vi "Main Host Comms Commands.vi"(8 "error in":errorcluster, 10 "main queue":refnum<queue>, 11 "tcp in":refnum<k5>) -> (0 "error out":errorcluster, 2 "processed?":bool, 3 "tcp out":refnum<k5>)   [LabVIEW 2019]
uses:
  RT Controls/Main Process Commands.ctl
  RT Controls/Main Command Events.ctl
panel:
  out "error msg":string
  out "cmd":string
  out "subcmd":string
  out "full cmd":string
  out "single cmd?":bool
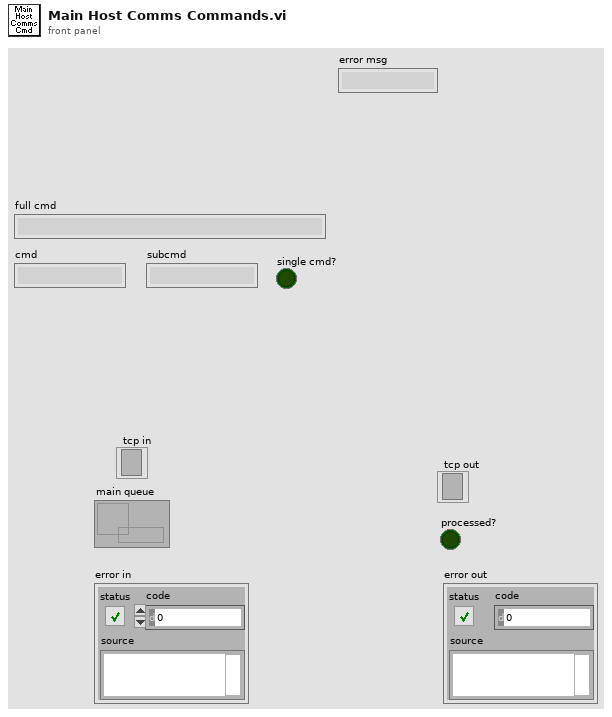
[diagram p1: front panel]
types:
  T1 = enum16{"Standard", "Buffered", "CRLF", "Immediate"}
  T2 = typedef "Main Process Commands.ctl" = cluster{"Commands":T3, "Value":variant}
  T3 = typedef "Main Command Events.ctl" = enum16{"Idle", "FullStop", "MainReadConfig", "MainWriteConfig", "OpenUpper", "CloseUpper", "OpenLower", "CloseLower", "SetWatchdogInt", "EnCloudShutDn", "DisCloudShutDn", "SetRainDelay", "EnAutoShutDn", "DisAutoShutDn", "SetRevDelay", "RotToAz", "RotLeft", "RotRight", "RotToHome", "DefineHomePos", "SetHSThres", "SetEncCounts", "SyncClose", "SyncOpen", "SetAZTimLim", "SetAZTol", "AZEncPositive", "AZEncNegative", "RotToCenter"}
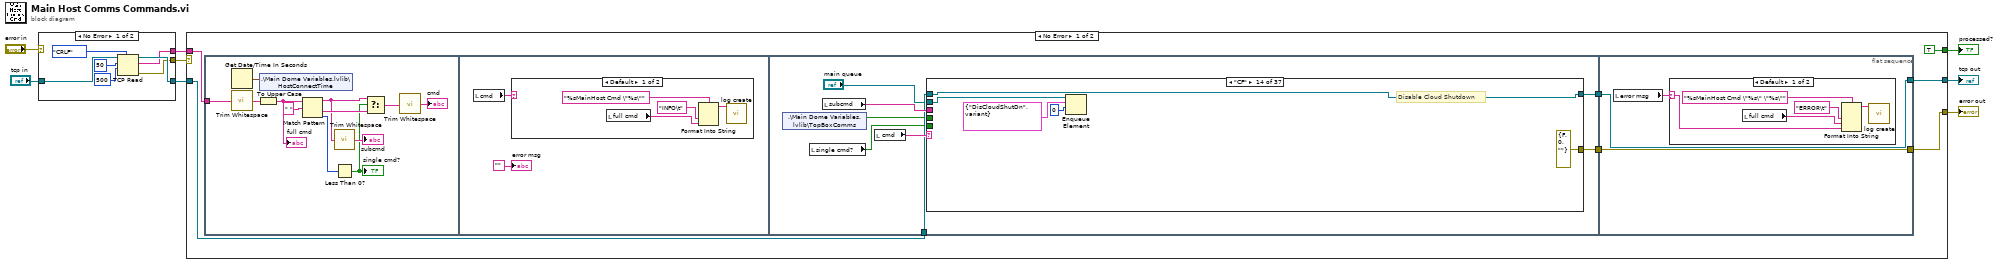
[diagram p0: block diagram]
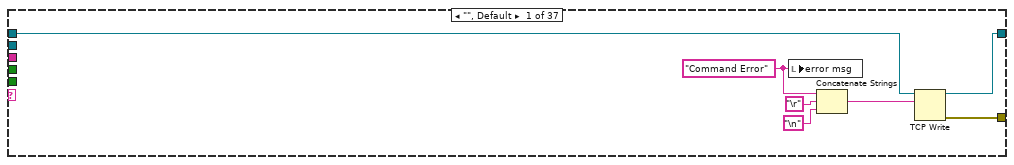
[diagram p3: hidden frame]
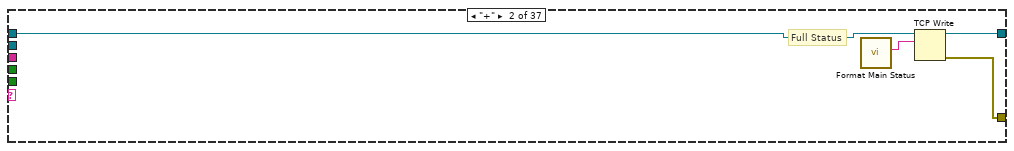
[diagram p4: hidden frame]
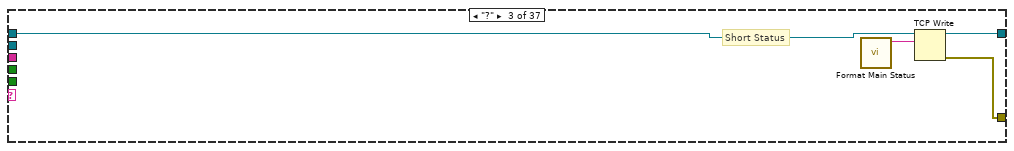
[diagram p5: hidden frame]
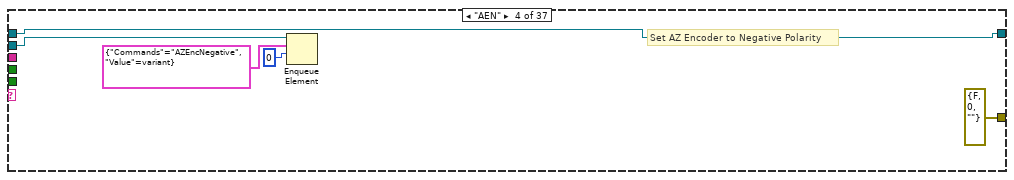
[diagram p6: hidden frame]
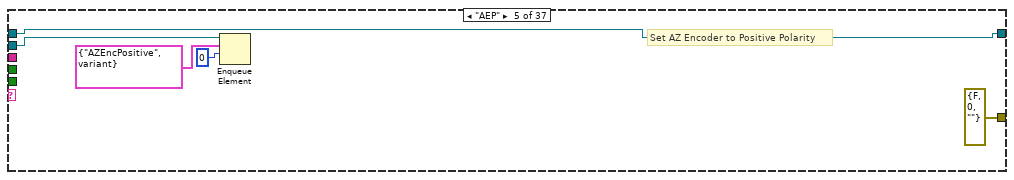
[diagram p7: hidden frame]
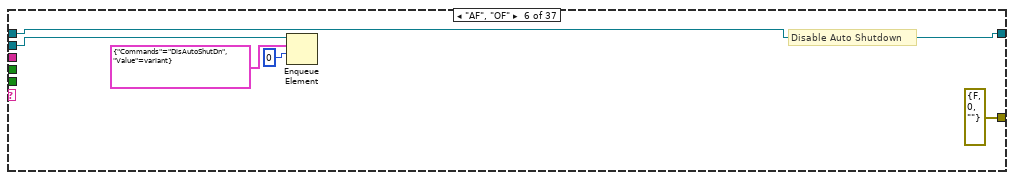
[diagram p8: hidden frame]
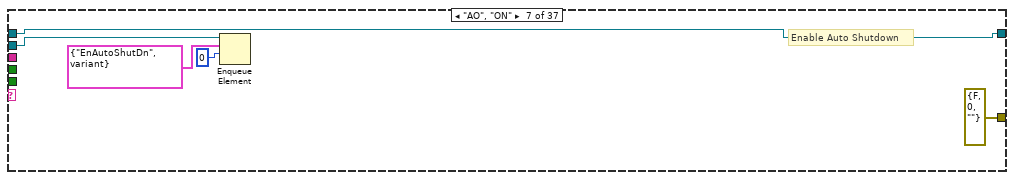
[diagram p9: hidden frame]
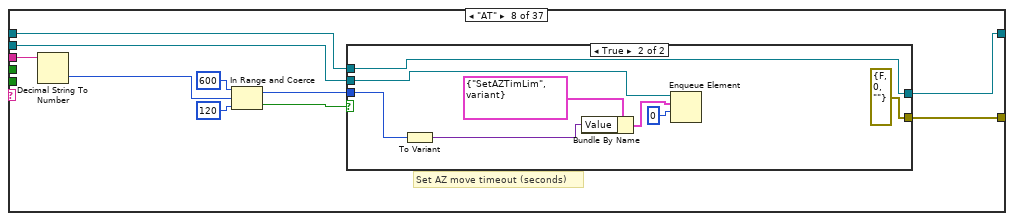
[diagram p10: hidden frame]
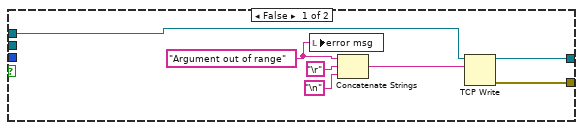
[diagram p11: hidden frame]
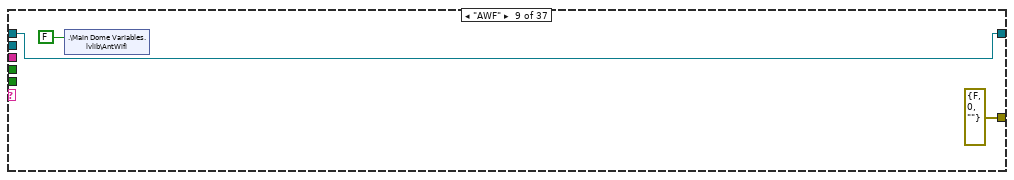
[diagram p12: hidden frame]
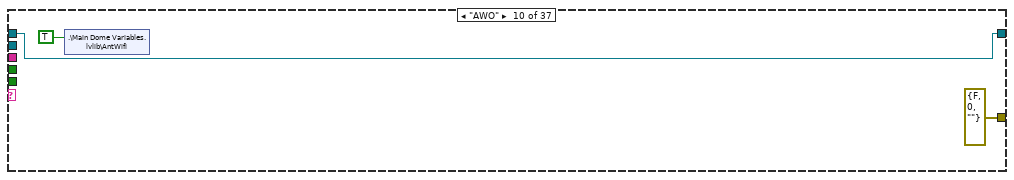
[diagram p13: hidden frame]
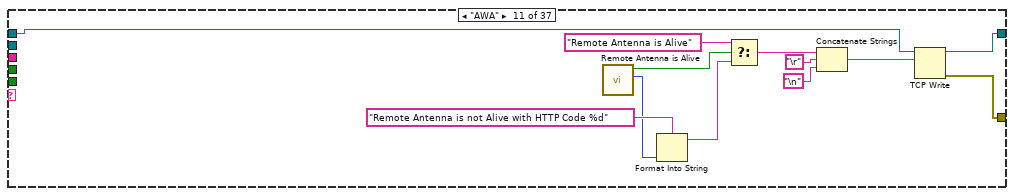
[diagram p14: hidden frame]
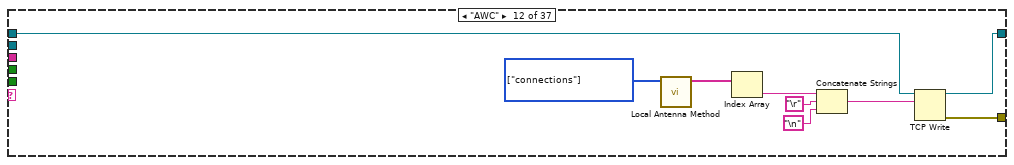
[diagram p15: hidden frame]
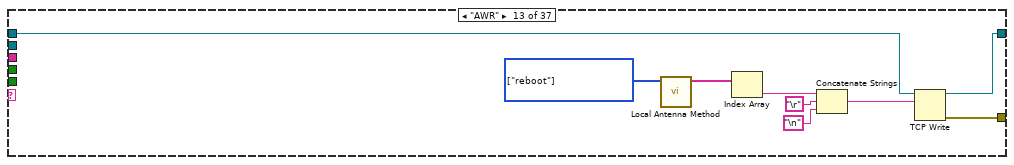
[diagram p16: hidden frame]
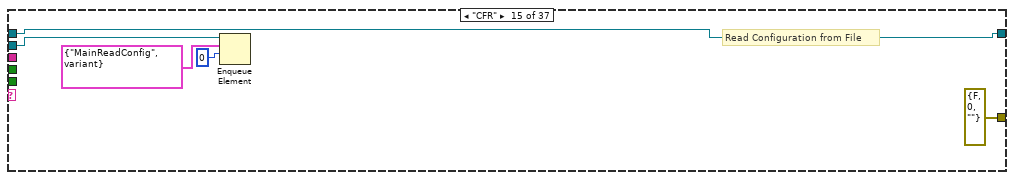
[diagram p17: hidden frame]
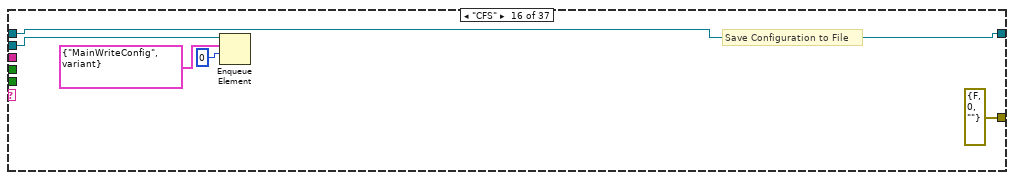
[diagram p18: hidden frame]
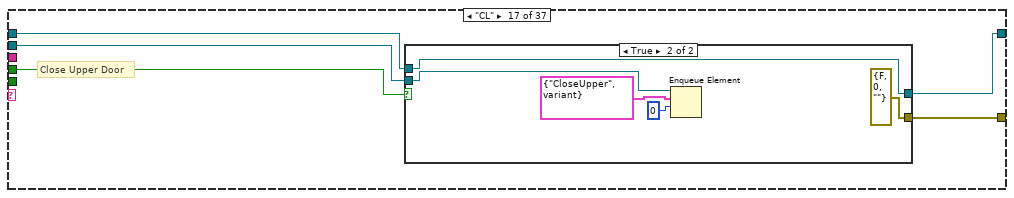
[diagram p19: hidden frame]
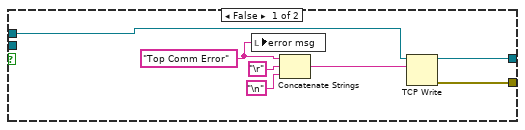
[diagram p20: hidden frame]
diagram:
  n1 = case shown="No Error" "error in" {
    selector: "error in" -> [_ w16]
    tunnel: "tcp in" -> [w15 w18]
    tunnel: [w11 w18] -> w6
    tunnel: [w10 "" ("data out")] -> w7
    tunnel: [w9 w16] -> w8
    frame No Error {
      n2 = TCP Read(connection ID=w15, bytes to read=50, 7:T1."CRLF" ("mode (standard)"), 9:500 ("timeout ms (25000)")) -> (connection ID out=w11:refnum<k5>, data out=w10:string, error out=w9:errorcluster)  [unwired: 1 in]
    }
    frame Error {
    }
  }
  n3 = case shown="No Error" w8 {
    selector: w8 -> [_ w570]
    tunnel: w7 -> [w24 _]
    tunnel: w6 -> [w23 w567]
    tunnel: [w21 w567] -> w2
    tunnel: [w22 w569] -> w3
    tunnel: [TRUE FALSE] -> w1
    frame No Error {
      n4 = flat-sequence {
        tunnel: w24 -> [w28]
        tunnel: w23 -> [w49]
        tunnel: [w48] -> w20
        tunnel: [w47] -> w19
        tunnel: [w560] -> w21
        tunnel: [w561] -> w22
        tunnel: w20 -> [w561]
        tunnel: w19 -> [w560]
        frame #0 {
          n5 = Get Date/Time In Seconds() -> (seconds since 1Jan1904=w26:timestamp)
          n6 = call <vilib>:"Trim Whitespace.vi"("string"=w28) -> ("trimmed string"=w37:string)  [unwired: 1 in]
          n7 = To Upper Case(1:w37) -> (0:w27:string)
          "full cmd" <- w27
          n8 = shared-variable ".\\Main Dome Variables.lvlib\\HostConnectTime"(w26) -> ()  [unwired: 1 in, 1 out]
          n9 = Match Pattern(string=w27, regular expression=" ") -> (before substring=w31:string, after substring=w34:string, offset past match=w35:i32)  [unwired: 1 in, 1 out]
          n10 = call <vilib>:"Trim Whitespace.vi"("string"=w31) -> ("trimmed string"=→"subcmd":string)  [unwired: 1 in]
          n11 = Less Than 0?(x=w35) -> (x < 0?=w29:bool)
          "single cmd?" <- w29
          n12 = Select(t=w31, s=w29, f=w34) -> (s? t:f=w32:string)
          n13 = call <vilib>:"Trim Whitespace.vi"("string"=w32) -> ("trimmed string"=→"cmd":string)  [unwired: 1 in]
        }
        frame #1 {
          n14 = local read "cmd"() -> (w39:string)
          n15 = case shown="Default" w39 {
            frame Default {
              n16 = local read "full cmd"() -> (w40:string)
              n17 = Format Into String(format string="%sMainHost Cmd \"%s\"", "INFO\t" ("input 1"), w40) -> (resulting string=w41:string)  [unwired: 2 in, 1 out]
              n18 = call "log create.vi"("message"=w41) -> ()  [unwired: 11 in]
            }
            frame "+", "?", "HELP" {
            }
          }
          "error msg" <- ""
        }
        frame #2 {
          n19 = shared-variable ".\\Main Dome Variables.lvlib\\TopBoxComms"() -> (w46:bool)  [unwired: 1 in, 1 out]
          n20 = local read "single cmd?"() -> (w45:bool)
          n21 = local read "subcmd"() -> (w51:string)
          n22 = local read "cmd"() -> (w50:string)
          n23 = case shown="\"CF\"" w50 {
            tunnel: w49 -> [w56 w60 w65 w71 w76 w81 w86 w93 w112 w115 w126 w132 w141 w152 w157 w162 w167 w184 w189 w193 w210 w215 w225 w253 w281 w311 w337 w359 w383 w405 w435 w457 w475 w491 w504 w524 w541]
            tunnel: [w58 w62 w66 errorcluster {"status"=FALSE, "code"=0, "source"=""} ("error out") errorcluster {"status"=FALSE, "code"=0, "source"=""} ("error out") errorcluster {"status"=FALSE, "code"=0, "source"=""} ("error out") errorcluster {"status"=FALSE, "code"=0, "source"=""} ("error out") w89 errorcluster {"status"=FALSE, "code"=0, "source"=""} ("error out") errorcluster {"status"=FALSE, "code"=0, "source"=""} ("error out") w118 w130 w139 errorcluster {"status"=FALSE, "code"=0, "source"=""} ("error out") errorcluster {"status"=FALSE, "code"=0, "source"=""} ("error out") errorcluster {"status"=FALSE, "code"=0, "source"=""} ("error out") w164 errorcluster {"status"=FALSE, "code"=0, "source"=""} ("error out") errorcluster {"status"=FALSE, "code"=0, "source"=""} ("error out") w192 w208 errorcluster {"status"=FALSE, "code"=0, "source"=""} ("error out") w222 w250 w279 w309 w334 w358 w380 w404 w432 w455 w472 errorcluster {"status"=FALSE, "code"=0, "source"=""} ("error out") w502 w522 w540] -> w48
            tunnel: [w57 w61 w64 w71 w76 w81 w86 w90 w112 w115 w125 w131 w140 w152 w157 w162 w165 w184 w189 w191 w209 w215 w223 w251 w280 w310 w335 w357 w381 w403 w433 w456 w473 w491 w503 w521 w539] -> w47
            tunnel: w51 -> [_ _ _ _ _ _ _ w92 _ _ _ _ _ _ _ _ _ _ _ _ _ _ w221 w249 w278 w304 w333 _ w379 w410 w431 _ _ _ w497 _ w543]
            tunnel: w45 -> [_ _ _ _ _ _ _ _ _ _ _ _ _ _ _ _ _ _ _ _ _ _ w218 w246 w274 w301 w330 _ w376 _ w428 _ _ _ w494 _ _]
            tunnel: w46 -> [_ _ _ _ _ _ _ _ _ _ _ _ _ _ _ _ w166 _ _ w194 _ _ _ _ _ _ _ w360 _ _ _ w458 w474 _ _ w523 _]
            tunnel: "main queue" -> [_ _ _ w68 w73 w78 w83 w87 _ _ _ _ _ w148 w154 w159 w163 w181 w186 w190 _ w212 w217 w245 w273 w300 w329 w356 w375 w401 w427 w454 w471 w490 w493 w520 w537]
            frame "", Default {
              w52 = "Command Error" ("data in")
              n24 = local write "error msg"(w52) -> ()
              n25 = Concatenate Strings(w52, "\r", "\n") -> (w53:string)
              n26 = TCP Write(connection ID=w56, data in=w53) -> (connection ID out=w57:refnum<k5>, error out=w58:errorcluster)  [unwired: 2 in, 1 out]
            }
            frame "+" {
              # "Full Status"
              n27 = call "Format Main Status.vi"() -> ("FullStat"=w59:string)  [unwired: 10 in, 1 out]
              n28 = TCP Write(connection ID=w60, data in=w59) -> (connection ID out=w61:refnum<k5>, error out=w62:errorcluster)  [unwired: 2 in, 1 out]
            }
            frame "?" {
              # "Short Status"
              n29 = call "Format Main Status.vi"() -> ("ShortStat"=w63:string)  [unwired: 10 in, 1 out]
              n30 = TCP Write(connection ID=w65, data in=w63) -> (connection ID out=w64:refnum<k5>, error out=w66:errorcluster)  [unwired: 2 in, 1 out]
            }
            frame "AEN" {
              # "Set AZ Encoder to Negative Polarity"
              n31 = Enqueue Element(queue=w68, element=T2 {"Commands"=enum."AZEncNegative", "Value"=variant} ("event data"), timeout in ms (-1)=0) -> ()  [unwired: 1 in, 3 out]
            }
            frame "AEP" {
              # "Set AZ Encoder to Positive Polarity"
              n32 = Enqueue Element(queue=w73, element=T2 {"Commands"=enum."AZEncPositive", "Value"=variant} ("event data"), timeout in ms (-1)=0) -> ()  [unwired: 1 in, 3 out]
            }
            frame "AF", "OF" {
              # "Disable Auto Shutdown"
              n33 = Enqueue Element(queue=w78, element=T2 {"Commands"=enum."DisAutoShutDn", "Value"=variant} ("event data"), timeout in ms (-1)=0) -> ()  [unwired: 1 in, 3 out]
            }
            frame "AO", "ON" {
              # "Enable Auto Shutdown"
              n34 = Enqueue Element(queue=w83, element=T2 {"Commands"=enum."EnAutoShutDn", "Value"=variant} ("event data"), timeout in ms (-1)=0) -> ()  [unwired: 1 in, 3 out]
            }
            frame "AT" {
              # "Set AZ move timeout (seconds)"
              n35 = Decimal String To Number(string=w92) -> (number=w96:i32)  [unwired: 2 in, 1 out]
              n36 = In Range and Coerce(upper limit=600, x=w96, lower limit=120) -> (coerced(x)=w91:i32, In Range?=w94:bool)
              n37 = case shown="True" w94 {
                tunnel: w93 -> [w102 w111]
                tunnel: [w103 errorcluster {"status"=FALSE, "code"=0, "source"=""} ("error out")] -> w89
                tunnel: [w101 w111] -> w90
                tunnel: w91 -> [_ w110]
                tunnel: w87 -> [_ w105]
                frame False {
                  w97 = "Argument out of range" ("data in")
                  n38 = local write "error msg"(w97) -> ()
                  n39 = Concatenate Strings(w97, "\r", "\n") -> (w98:string)
                  n40 = TCP Write(connection ID=w102, data in=w98) -> (connection ID out=w101:refnum<k5>, error out=w103:errorcluster)  [unwired: 2 in, 1 out]
                }
                frame True {
                  n41 = To Variant(anything=w110) -> (Variant=w109:variant)
                  n42 = Bundle By Name(cluster=T2 {"Commands"=enum."SetAZTimLim", "Value"=variant} ("event data"), "Value"=w109) -> (w106:T2)
                  n43 = Enqueue Element(queue=w105, element=w106, timeout in ms (-1)=0) -> ()  [unwired: 1 in, 3 out]
                }
              }
            }
            frame "AWF" {
              n44 = shared-variable ".\\Main Dome Variables.lvlib\\AntWifi"(FALSE ("AntWifi")) -> ()  [unwired: 1 in, 1 out]
            }
            frame "AWO" {
              n45 = shared-variable ".\\Main Dome Variables.lvlib\\AntWifi"(TRUE ("AntWifi")) -> ()  [unwired: 1 in, 1 out]
            }
            frame "AWA" {
              n46 = call "Remote Antenna is Alive.vi"() -> ("http code"=w120:i32, "alive?"=w124:bool)  [unwired: 10 in]
              n47 = Format Into String(format string="Remote Antenna is not Alive with HTTP Code %d", w120) -> (resulting string=w119:string)  [unwired: 2 in, 1 out]
              n48 = Select(t="Remote Antenna is Alive" ("data in"), s=w124, f=w119) -> (s? t:f=w122:string)
              n49 = Concatenate Strings(w122, "\r", "\n") -> (w129:string)
              n50 = TCP Write(connection ID=w126, data in=w129) -> (connection ID out=w125:refnum<k5>, error out=w118:errorcluster)  [unwired: 2 in, 1 out]
            }
            frame "AWC" {
              w138 = enum16{"connections", "reboot"}[] [enum."connections"] items=["connections", "reboot"] ("command (connections)")
              n51 = call "Local Antenna Method.vi"("command"=w138) -> ("out"=w137:string[])  [unwired: 10 in]
              n52 = Index Array(array=w137) -> (element=w133:string)  [unwired: 1 in]
              n53 = Concatenate Strings(w133, "\r", "\n") -> (w136:string)
              n54 = TCP Write(connection ID=w132, data in=w136) -> (connection ID out=w131:refnum<k5>, error out=w130:errorcluster)  [unwired: 2 in, 1 out]
            }
            frame "AWR" {
              w142 = enum16{"connections", "reboot"}[] [enum."reboot"] items=["connections", "reboot"] ("command (connections)")
              n55 = call "Local Antenna Method.vi"("command"=w142) -> ("out"=w147:string[])  [unwired: 10 in]
              n56 = Index Array(array=w147) -> (element=w145:string)  [unwired: 1 in]
              n57 = Concatenate Strings(w145, "\r", "\n") -> (w146:string)
              n58 = TCP Write(connection ID=w141, data in=w146) -> (connection ID out=w140:refnum<k5>, error out=w139:errorcluster)  [unwired: 2 in, 1 out]
            }
            frame "CF" {
              # "Disable Cloud Shutdown"
              n59 = Enqueue Element(queue=w148, element=T2 {"Commands"=enum."DisCloudShutDn", "Value"=variant} ("event data"), timeout in ms (-1)=0) -> ()  [unwired: 1 in, 3 out]
            }
            frame "CFR" {
              # "Read Configuration from File"
              n60 = Enqueue Element(queue=w154, element=T2 {"Commands"=enum."MainReadConfig", "Value"=variant} ("event data"), timeout in ms (-1)=0) -> ()  [unwired: 1 in, 3 out]
            }
            frame "CFS" {
              # "Save Configuration to File"
              n61 = Enqueue Element(queue=w159, element=T2 {"Commands"=enum."MainWriteConfig", "Value"=variant} ("event data"), timeout in ms (-1)=0) -> ()  [unwired: 1 in, 3 out]
            }
            frame "CL" {
              # "Close Upper Door"
              n62 = case shown="True" w166 {
                tunnel: w167 -> [w170 w179]
                tunnel: [w169 w179] -> w165
                tunnel: [w171 errorcluster {"status"=FALSE, "code"=0, "source"=""} ("error out")] -> w164
                tunnel: w163 -> [_ w176]
                frame False {
                  w168 = "Top Comm Error" ("data in")
                  n63 = local write "error msg"(w168) -> ()
                  n64 = Concatenate Strings(w168, "\r", "\n") -> (w172:string)
                  n65 = TCP Write(connection ID=w170, data in=w172) -> (connection ID out=w169:refnum<k5>, error out=w171:errorcluster)  [unwired: 2 in, 1 out]
                }
                frame True {
                  n66 = Enqueue Element(queue=w176, element=T2 {"Commands"=enum."CloseUpper", "Value"=variant} ("event data"), timeout in ms (-1)=0) -> ()  [unwired: 1 in, 3 out]
                }
              }
            }
            frame "CN" {
              # "Send Dome to Encoder Center"
              n67 = Enqueue Element(queue=w181, element=T2 {"Commands"=enum."RotToCenter", "Value"=variant} ("event data"), timeout in ms (-1)=0) -> ()  [unwired: 1 in, 3 out]
            }
            frame "CO" {
              # "Enable Cloud Shutdown"
              n68 = Enqueue Element(queue=w186, element=T2 {"Commands"=enum."EnCloudShutDn", "Value"=variant} ("event data"), timeout in ms (-1)=0) -> ()  [unwired: 1 in, 3 out]
            }
            frame "DN" {
              # "Open Lower Door"
              n69 = case shown="False" w194 {
                tunnel: w193 -> [w196 w206]
                tunnel: [w198 errorcluster {"status"=FALSE, "code"=0, "source"=""} ("error out")] -> w192
                tunnel: [w197 w206] -> w191
                tunnel: w190 -> [_ w202]
                frame False {
                  w195 = "Top Comm Error" ("data in")
                  n70 = local write "error msg"(w195) -> ()
                  n71 = Concatenate Strings(w195, "\r", "\n") -> (w199:string)
                  n72 = TCP Write(connection ID=w196, data in=w199) -> (connection ID out=w197:refnum<k5>, error out=w198:errorcluster)  [unwired: 2 in, 1 out]
                }
                frame True {
                  n73 = Enqueue Element(queue=w202, element=T2 {"Commands"=enum."OpenLower", "Value"=variant} ("event data"), timeout in ms (-1)=0) -> ()  [unwired: 1 in, 3 out]
                }
              }
            }
            frame "HELP" {
              n74 = call "Host Help Text.vi"() -> ("Help Text"=w207:string)  [unwired: 11 in]
              n75 = TCP Write(connection ID=w210, data in=w207) -> (connection ID out=w209:refnum<k5>, error out=w208:errorcluster)  [unwired: 2 in, 1 out]
            }
            frame "HM" {
              # "Send Dome to Home"
              n76 = Enqueue Element(queue=w212, element=T2 {"Commands"=enum."RotToHome", "Value"=variant} ("event data"), timeout in ms (-1)=0) -> ()  [unwired: 1 in, 3 out]
            }
            frame "HS" {
              # "Set High Speed Threshold (deg)"
              n77 = Fract/Exp String To Number(string=w221, default (0 dbl)=-10.0 ("default (0 DBL)")) -> (number=w228:dbl)  [unwired: 2 in, 1 out]
              n78 = In Range and Coerce(upper limit=10.0, x=w228, lower limit=0.0) -> (coerced(x)=w224:dbl, In Range?=w220:bool)
              n79 = Compound Arithmetic op=AND(invert w218, w220) -> (w219:bool)
              n80 = case shown="True" w219 {
                tunnel: w225 -> [w234 w243]
                tunnel: [w235 errorcluster {"status"=FALSE, "code"=0, "source"=""} ("error out")] -> w222
                tunnel: [w233 w243] -> w223
                tunnel: w224 -> [_ w242]
                tunnel: w217 -> [_ w237]
                frame False {
                  w229 = "Argument out of range" ("data in")
                  n81 = local write "error msg"(w229) -> ()
                  n82 = Concatenate Strings(w229, "\r", "\n") -> (w230:string)
                  n83 = TCP Write(connection ID=w234, data in=w230) -> (connection ID out=w233:refnum<k5>, error out=w235:errorcluster)  [unwired: 2 in, 1 out]
                }
                frame True {
                  n84 = To Variant(anything=w242) -> (Variant=w241:variant)
                  n85 = Bundle By Name(cluster=T2 {"Commands"=enum."SetHSThres", "Value"=variant} ("event data"), "Value"=w241) -> (w238:T2)
                  n86 = Enqueue Element(queue=w237, element=w238, timeout in ms (-1)=0) -> ()  [unwired: 1 in, 3 out]
                }
              }
            }
            frame "HZ" {
              # "Define Dome Home Position (degs)"
              n87 = Fract/Exp String To Number(string=w249, default (0 dbl)=-10.0 ("lower limit")) -> (number=w256:dbl)  [unwired: 2 in, 1 out]
              n88 = In Range and Coerce(upper limit=360.0, x=w256, lower limit=0.0) -> (coerced(x)=w252:dbl, In Range?=w247:bool)
              n89 = Compound Arithmetic op=AND(invert w246, w247) -> (w248:bool)
              n90 = case shown="True" w248 {
                tunnel: w253 -> [w262 w271]
                tunnel: [w263 errorcluster {"status"=FALSE, "code"=0, "source"=""} ("error out")] -> w250
                tunnel: [w261 w271] -> w251
                tunnel: w252 -> [_ w270]
                tunnel: w245 -> [_ w265]
                frame False {
                  w257 = "Argument out of range" ("data in")
                  n91 = local write "error msg"(w257) -> ()
                  n92 = Concatenate Strings(w257, "\r", "\n") -> (w258:string)
                  n93 = TCP Write(connection ID=w262, data in=w258) -> (connection ID out=w261:refnum<k5>, error out=w263:errorcluster)  [unwired: 2 in, 1 out]
                }
                frame True {
                  n94 = To Variant(anything=w270) -> (Variant=w269:variant)
                  n95 = Bundle By Name(cluster=T2 {"Commands"=enum."DefineHomePos", "Value"=variant} ("event data"), "Value"=w269) -> (w266:T2)
                  n96 = Enqueue Element(queue=w265, element=w266, timeout in ms (-1)=0) -> ()  [unwired: 1 in, 3 out]
                }
              }
            }
            frame "LF" {
              # "Rotate Dome Left by Degrees"
              n97 = Fract/Exp String To Number(string=w278, default (0 dbl)=-10.0 ("default (0 DBL)")) -> (number=w284:dbl)  [unwired: 2 in, 1 out]
              n98 = In Range and Coerce(upper limit=360.0, x=w284, lower limit=0.0) -> (coerced(x)=w277:dbl, In Range?=w276:bool)
              n99 = Compound Arithmetic op=AND(invert w274, w276) -> (w275:bool)
              n100 = case shown="True" w275 {
                tunnel: w281 -> [w290 w299]
                tunnel: [w291 errorcluster {"status"=FALSE, "code"=0, "source"=""} ("error out")] -> w279
                tunnel: [w289 w299] -> w280
                tunnel: w277 -> [_ w298]
                tunnel: w273 -> [_ w292]
                frame False {
                  w285 = "Argument out of range" ("data in")
                  n101 = local write "error msg"(w285) -> ()
                  n102 = Concatenate Strings(w285, "\r", "\n") -> (w286:string)
                  n103 = TCP Write(connection ID=w290, data in=w286) -> (connection ID out=w289:refnum<k5>, error out=w291:errorcluster)  [unwired: 2 in, 1 out]
                }
                frame True {
                  n104 = To Variant(anything=w298) -> (Variant=w297:variant)
                  n105 = Bundle By Name(cluster=T2 {"Commands"=enum."RotLeft", "Value"=variant} ("event data"), "Value"=w297) -> (w293:T2)
                  n106 = Enqueue Element(queue=w292, element=w293, timeout in ms (-1)=0) -> ()  [unwired: 1 in, 3 out]
                }
              }
            }
            frame "LM" {
              # "Set Encoder Counts in 360 deg"
              n107 = Fract/Exp String To Number(string=w304) -> (number=w308:dbl)  [unwired: 3 in, 1 out]
              n108 = In Range and Coerce(upper limit=inf, x=w308, lower limit=1.0) -> (coerced(x)=w305:dbl, In Range?=w303:bool)
              n109 = Compound Arithmetic op=AND(invert w301, w303) -> (w302:bool)
              n110 = case shown="True" w302 {
                tunnel: w311 -> [w317 w327]
                tunnel: [w318 errorcluster {"status"=FALSE, "code"=0, "source"=""} ("error out")] -> w309
                tunnel: [w316 w327] -> w310
                tunnel: w305 -> [_ w320]
                tunnel: w300 -> [_ w322]
                frame False {
                  w312 = "Argument out of range" ("data in")
                  n111 = local write "error msg"(w312) -> ()
                  n112 = Concatenate Strings(w312, "\r", "\n") -> (w313:string)
                  n113 = TCP Write(connection ID=w317, data in=w313) -> (connection ID out=w316:refnum<k5>, error out=w318:errorcluster)  [unwired: 2 in, 1 out]
                }
                frame True {
                  n114 = To Unsigned Quad Integer(1:w320) -> (0:w319:u64)
                  n115 = To Variant(anything=w319) -> (Variant=w326:variant)
                  n116 = Bundle By Name(cluster=T2 {"Commands"=enum."SetEncCounts", "Value"=variant} ("event data"), "Value"=w326) -> (w323:T2)
                  n117 = Enqueue Element(queue=w322, element=w323, timeout in ms (-1)=0) -> ()  [unwired: 1 in, 3 out]
                }
              }
            }
            frame "MV" {
              # "Rotate Dome to Az Position (deg)"
              n118 = Fract/Exp String To Number(string=w333, default (0 dbl)=-10.0 ("default (0 DBL)")) -> (number=w340:dbl)  [unwired: 2 in, 1 out]
              n119 = In Range and Coerce(upper limit=360.0, x=w340, lower limit=0.0) -> (coerced(x)=w336:dbl, In Range?=w332:bool)
              n120 = Compound Arithmetic op=AND(invert w330, w332) -> (w331:bool)
              n121 = case shown="True" w331 {
                tunnel: w337 -> [w346 w355]
                tunnel: [w347 errorcluster {"status"=FALSE, "code"=0, "source"=""} ("error out")] -> w334
                tunnel: [w345 w355] -> w335
                tunnel: w336 -> [_ w354]
                tunnel: w329 -> [_ w348]
                frame False {
                  w341 = "Argument out of range" ("data in")
                  n122 = local write "error msg"(w341) -> ()
                  n123 = Concatenate Strings(w341, "\r", "\n") -> (w342:string)
                  n124 = TCP Write(connection ID=w346, data in=w342) -> (connection ID out=w345:refnum<k5>, error out=w347:errorcluster)  [unwired: 2 in, 1 out]
                }
                frame True {
                  n125 = To Variant(anything=w354) -> (Variant=w353:variant)
                  n126 = Bundle By Name(cluster=T2 {"Commands"=enum."RotToAz", "Value"=variant} ("event data"), "Value"=w353) -> (w349:T2)
                  n127 = Enqueue Element(queue=w348, element=w349, timeout in ms (-1)=0) -> ()  [unwired: 1 in, 3 out]
                }
              }
            }
            frame "OP" {
              # "Open Upper Door"
              n128 = case shown="True" w360 {
                tunnel: w359 -> [w362 w372]
                tunnel: [w364 errorcluster {"status"=FALSE, "code"=0, "source"=""} ("error out")] -> w358
                tunnel: [w363 w372] -> w357
                tunnel: w356 -> [_ w369]
                frame False {
                  w361 = "Top Comm Error" ("data in")
                  n129 = local write "error msg"(w361) -> ()
                  n130 = Concatenate Strings(w361, "\r", "\n") -> (w365:string)
                  n131 = TCP Write(connection ID=w362, data in=w365) -> (connection ID out=w363:refnum<k5>, error out=w364:errorcluster)  [unwired: 2 in, 1 out]
                }
                frame True {
                  n132 = Enqueue Element(queue=w369, element=T2 {"Commands"=enum."OpenUpper", "Value"=variant} ("event data"), timeout in ms (-1)=0) -> ()  [unwired: 1 in, 3 out]
                }
              }
            }
            frame "RD" {
              # "Set Reverse Direction Delay (s)"
              n133 = Decimal String To Number(string=w379, default (0L)=-10 ("default (0 I32)")) -> (number=w374:i32)  [unwired: 1 in, 1 out]
              n134 = In Range and Coerce(upper limit=6, x=w374, lower limit=0) -> (coerced(x)=w382:i32, In Range?=w377:bool)
              n135 = Compound Arithmetic op=AND(invert w376, w377) -> (w378:bool)
              n136 = case shown="True" w378 {
                tunnel: w383 -> [w391 w400]
                tunnel: [w392 errorcluster {"status"=FALSE, "code"=0, "source"=""} ("error out")] -> w380
                tunnel: [w390 w400] -> w381
                tunnel: w382 -> [_ w399]
                tunnel: w375 -> [_ w394]
                frame False {
                  w386 = "Argument out of range" ("data in")
                  n137 = local write "error msg"(w386) -> ()
                  n138 = Concatenate Strings(w386, "\r", "\n") -> (w387:string)
                  n139 = TCP Write(connection ID=w391, data in=w387) -> (connection ID out=w390:refnum<k5>, error out=w392:errorcluster)  [unwired: 2 in, 1 out]
                }
                frame True {
                  n140 = To Variant(anything=w399) -> (Variant=w398:variant)
                  n141 = Bundle By Name(cluster=T2 {"Commands"=enum."SetRevDelay", "Value"=variant} ("event data"), "Value"=w398) -> (w395:T2)
                  n142 = Enqueue Element(queue=w394, element=w395, timeout in ms (-1)=0) -> ()  [unwired: 1 in, 3 out]
                }
              }
            }
            frame "RS" {
              # "Set Rain/Snow Activate Delay"
              n143 = Decimal String To Number(string=w410) -> (number=w409:i32)  [unwired: 2 in, 1 out]
              n144 = In Range and Coerce(upper limit=10, x=w409, lower limit=1) -> (coerced(x)=w402:i32, In Range?=w406:bool)
              n145 = case shown="True" w406 {
                tunnel: w405 -> [w415 w425]
                tunnel: [w417 errorcluster {"status"=FALSE, "code"=0, "source"=""} ("error out")] -> w404
                tunnel: [w416 w425] -> w403
                tunnel: w402 -> [_ w423]
                tunnel: w401 -> [_ w419]
                frame False {
                  w411 = "Invalid Argument" ("data in")
                  n146 = local write "error msg"(w411) -> ()
                  n147 = Concatenate Strings(w411, "\r", "\n") -> (w412:string)
                  n148 = TCP Write(connection ID=w415, data in=w412) -> (connection ID out=w416:refnum<k5>, error out=w417:errorcluster)  [unwired: 2 in, 1 out]
                }
                frame True {
                  n149 = To Variant(anything=w423) -> (Variant=w422:variant)
                  n150 = Bundle By Name(cluster=T2 {"Commands"=enum."SetRainDelay", "Value"=variant} ("event data"), "Value"=w422) -> (w420:T2)
                  n151 = Enqueue Element(queue=w419, element=w420, timeout in ms (-1)=0) -> ()  [unwired: 1 in, 3 out]
                }
              }
            }
            frame "RT" {
              # "Rotate Dome Right by Degrees"
              n152 = Fract/Exp String To Number(string=w431, default (0 dbl)=-10.0 ("default (0 DBL)")) -> (number=w438:dbl)  [unwired: 2 in, 1 out]
              n153 = In Range and Coerce(upper limit=360.0, x=w438, lower limit=0.0) -> (coerced(x)=w434:dbl, In Range?=w430:bool)
              n154 = Compound Arithmetic op=AND(invert w428, w430) -> (w429:bool)
              n155 = case shown="True" w429 {
                tunnel: w435 -> [w444 w453]
                tunnel: [w445 errorcluster {"status"=FALSE, "code"=0, "source"=""} ("error out")] -> w432
                tunnel: [w443 w453] -> w433
                tunnel: w434 -> [_ w452]
                tunnel: w427 -> [_ w447]
                frame False {
                  w439 = "Argument out of range" ("data in")
                  n156 = local write "error msg"(w439) -> ()
                  n157 = Concatenate Strings(w439, "\r", "\n") -> (w440:string)
                  n158 = TCP Write(connection ID=w444, data in=w440) -> (connection ID out=w443:refnum<k5>, error out=w445:errorcluster)  [unwired: 2 in, 1 out]
                }
                frame True {
                  n159 = To Variant(anything=w452) -> (Variant=w451:variant)
                  n160 = Bundle By Name(cluster=T2 {"Commands"=enum."RotRight", "Value"=variant} ("event data"), "Value"=w451) -> (w448:T2)
                  n161 = Enqueue Element(queue=w447, element=w448, timeout in ms (-1)=0) -> ()  [unwired: 1 in, 3 out]
                }
              }
            }
            frame "SC" {
              # "Sync Close"
              n162 = case shown="True" w458 {
                tunnel: w457 -> [w460 w467]
                tunnel: [w461 w467] -> w456
                tunnel: [w462 errorcluster {"status"=FALSE, "code"=0, "source"=""} ("error out")] -> w455
                tunnel: w454 -> [_ w468]
                frame False {
                  w459 = "Top Comm Error" ("data in")
                  n163 = local write "error msg"(w459) -> ()
                  n164 = Concatenate Strings(w459, "\r", "\n") -> (w463:string)
                  n165 = TCP Write(connection ID=w460, data in=w463) -> (connection ID out=w461:refnum<k5>, error out=w462:errorcluster)  [unwired: 2 in, 1 out]
                }
                frame True {
                  n166 = Enqueue Element(queue=w468, element=T2 {"Commands"=enum."SyncClose", "Value"=variant} ("event data"), timeout in ms (-1)=0) -> ()  [unwired: 1 in, 3 out]
                }
              }
            }
            frame "SO" {
              # "Sync Open"
              n167 = case shown="True" w474 {
                tunnel: w475 -> [w477 w487]
                tunnel: [w478 w487] -> w473
                tunnel: [w479 errorcluster {"status"=FALSE, "code"=0, "source"=""} ("error out")] -> w472
                tunnel: w471 -> [_ w484]
                frame False {
                  w476 = "Top Comm Error" ("data in")
                  n168 = local write "error msg"(w476) -> ()
                  n169 = Concatenate Strings(w476, "\r", "\n") -> (w480:string)
                  n170 = TCP Write(connection ID=w477, data in=w480) -> (connection ID out=w478:refnum<k5>, error out=w479:errorcluster)  [unwired: 2 in, 1 out]
                }
                frame True {
                  n171 = Enqueue Element(queue=w484, element=T2 {"Commands"=enum."SyncOpen", "Value"=variant} ("event data"), timeout in ms (-1)=0) -> ()  [unwired: 1 in, 3 out]
                }
              }
            }
            frame "ST" {
              # "Full stop"
              n172 = Lossy Enqueue Element(queue=w490, element=T2 {"Commands"=enum."FullStop", "Value"=variant} ("event data")) -> ()  [unwired: 1 in, 4 out]
            }
            frame "TOL" {
              # "Set AZ Position Yolerance (deg)"
              n173 = Fract/Exp String To Number(string=w497, default (0 dbl)=-10.0 ("default (0 DBL)")) -> (number=w501:dbl)  [unwired: 2 in, 1 out]
              n174 = In Range and Coerce(upper limit=3.0, x=w501, lower limit=0.0) -> (coerced(x)=w499:dbl, In Range?=w496:bool)
              n175 = Compound Arithmetic op=AND(invert w494, w496) -> (w495:bool)
              n176 = case shown="True" w495 {
                tunnel: w504 -> [w510 w519]
                tunnel: [w511 errorcluster {"status"=FALSE, "code"=0, "source"=""} ("error out")] -> w502
                tunnel: [w509 w519] -> w503
                tunnel: w499 -> [_ w518]
                tunnel: w493 -> [_ w513]
                frame False {
                  w505 = "Argument out of range" ("data in")
                  n177 = local write "error msg"(w505) -> ()
                  n178 = Concatenate Strings(w505, "\r", "\n") -> (w506:string)
                  n179 = TCP Write(connection ID=w510, data in=w506) -> (connection ID out=w509:refnum<k5>, error out=w511:errorcluster)  [unwired: 2 in, 1 out]
                }
                frame True {
                  n180 = To Variant(anything=w518) -> (Variant=w517:variant)
                  n181 = Bundle By Name(cluster=T2 {"Commands"=enum."SetAZTol", "Value"=variant} ("event data"), "Value"=w517) -> (w514:T2)
                  n182 = Enqueue Element(queue=w513, element=w514, timeout in ms (-1)=0) -> ()  [unwired: 1 in, 3 out]
                }
              }
            }
            frame "UP" {
              # "Close Lower Door"
              n183 = case shown="True" w523 {
                tunnel: w524 -> [w526 w536]
                tunnel: [w528 errorcluster {"status"=FALSE, "code"=0, "source"=""} ("error out")] -> w522
                tunnel: [w527 w536] -> w521
                tunnel: w520 -> [_ w533]
                frame False {
                  w525 = "Top Comm Error" ("data in")
                  n184 = local write "error msg"(w525) -> ()
                  n185 = Concatenate Strings(w525, "\r", "\n") -> (w529:string)
                  n186 = TCP Write(connection ID=w526, data in=w529) -> (connection ID out=w527:refnum<k5>, error out=w528:errorcluster)  [unwired: 2 in, 1 out]
                }
                frame True {
                  n187 = Enqueue Element(queue=w533, element=T2 {"Commands"=enum."CloseLower", "Value"=variant} ("event data"), timeout in ms (-1)=0) -> ()  [unwired: 1 in, 3 out]
                }
              }
            }
            frame "WT" {
              # "Set Watchdog Timer Interval"
              n188 = Decimal String To Number(string=w543) -> (number=w542:i32)  [unwired: 2 in, 1 out]
              n189 = Greater Than 0?(x=w542) -> (x > 0?=w538:bool)
              n190 = case shown="True" w538 {
                tunnel: w542 -> [_ w556]
                tunnel: w541 -> [w549 w558]
                tunnel: [w550 errorcluster {"status"=FALSE, "code"=0, "source"=""} ("error out")] -> w540
                tunnel: [w548 w558] -> w539
                tunnel: w537 -> [_ w552]
                frame False {
                  w544 = "Invalid Argument" ("data in")
                  n191 = local write "error msg"(w544) -> ()
                  n192 = Concatenate Strings(w544, "\r", "\n") -> (w545:string)
                  n193 = TCP Write(connection ID=w549, data in=w545) -> (connection ID out=w548:refnum<k5>, error out=w550:errorcluster)  [unwired: 2 in, 1 out]
                }
                frame True {
                  n194 = To Variant(anything=w556) -> (Variant=w555:variant)
                  n195 = Bundle By Name(cluster=T2 {"Commands"=enum."SetWatchdogInt", "Value"=variant} ("event data"), "Value"=w555) -> (w553:T2)
                  n196 = Enqueue Element(queue=w552, element=w553, timeout in ms (-1)=0) -> ()  [unwired: 1 in, 3 out]
                }
              }
            }
          }
        }
        frame #3 {
          n197 = local read "error msg"() -> (w559:string)
          n198 = case shown="Default" w559 {
            selector: w559 -> [w562 _]
            frame Default {
              n199 = local read "full cmd"() -> (w566:string)
              n200 = Format Into String(format string="%sMainHost Cmd \"%s\" \"%s\"", "ERROR\t" ("input 1"), w566, w562) -> (resulting string=w565:string)  [unwired: 2 in, 1 out]
              n201 = call "log create.vi"("message"=w565) -> ()  [unwired: 11 in]
            }
            frame "" {
            }
          }
        }
      }
    }
    frame Error {
      n202 = call <vilib>:"Clear Errors.vi"("error in (no error)"=w570, "specific error code to clear (0: all)"=56) -> ("error out"=w569:errorcluster)  [unwired: 4 in, 1 out]
    }
  }
  "error out" <- w3
  "tcp out" <- w2
  "processed?" <- w1
